vi "FRCts20_Backend_Division_POST.vi"(6 "Message Attributes":T4, 8 "error in (no error)":errorcluster, 10 "Data":string, 11 "Engine_Refnums":T1) -> (0 "error out":errorcluster)   [LabVIEW 2014]
doc: "Creates a new division under a competition. Called by the division/team api, and expects a division location and competition name."
uses:
  Dependencies/Keyed Array/KeyedArray.ctl
  FRCts20_Backend_EngineRefnums.ctl
  INI_Accessor/FRCts20_Backend_INI Controller.lvclass
  Dependencies/AMC/_SubVIs/TypeDefs/Message Queue.ctl
  Dependencies/AMC/_SubVIs/TypeDefs/Message.ctl
  <vilib>/addons/database/Connection.llb/Conn ObjectReference.ctl
  FRCts20_Backend_FGVOperation.ctl
  FRCts20_Backend_API/FRCts20_Backend_API_Division.ctl
  FRCts20_Backend_API/FRCts20_Backend_API_SW.ctl
  FRCts20_Backend_API/FRCts20_Backend_API_Status.ctl
  FRCts20_Backend_Engine.lvlib
  FRCts20_Backend_API/FRCts20_Backend_API.lvlib
  Dependencies/Keyed Array/Tools_KeyedArray.lvlib
  Dependencies/AMC/AMC.lvlib
  <vilib>/addons/database/NI_Database_API.lvlib
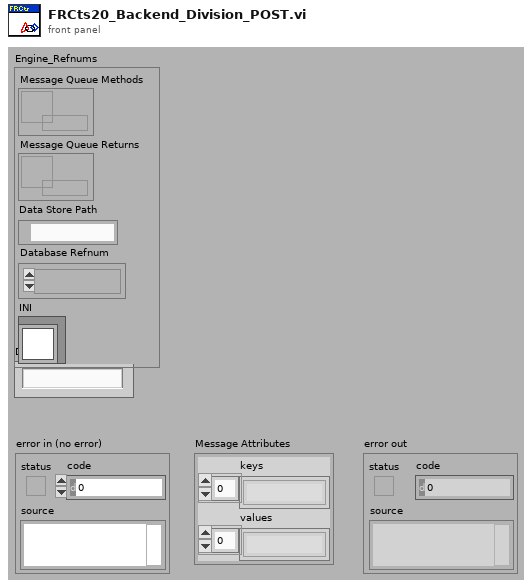
[diagram p1: front panel]
types:
  T1 = typedef "FRCts20_Backend_Engine.lvlib/FRCts20_Backend_EngineRefnums.ctl" = cluster{"Message Queue Methods":T2, "Message Queue Returns":T2, "Data Store Path":path, "Database Refnum":T3, "INI":refnum<class "FRCts20_Backend_INI Controller.lvclass">}
  T2 = typedef "AMC.lvlib/Message Queue.ctl" = refnum<queue>
  T3 = typedef "NI_Database_API.lvlib/Conn ObjectReference.ctl" = refnum<k1>
  T4 = typedef "Tools_KeyedArray.lvlib/KeyedArray.ctl" = cluster{"keys":string[], "values":string[]}
  T5 = typedef "FRCts20_Backend_API.lvlib/FRCts20_Backend_API_Division.ctl" = cluster{"Location":string, "Team":u32[], "APIReturn":string, "RootCmd":enum16{"Issues", "Software", "All"}, "SWType":T6, "Status":T7, "Competition":string}
  T6 = typedef "FRCts20_Backend_API.lvlib/FRCts20_Backend_API_SW.ctl" = string
  T7 = typedef "FRCts20_Backend_API.lvlib/FRCts20_Backend_API_Status.ctl" = enum16{"Open", "In Work", "Closed"}
  T8 = typedef "FRCts20_Backend_Engine.lvlib/FRCts20_Backend_FGVOperation.ctl" = enum16{"Initialize", "EnqueueMessage", "EnqueueDataReturn", "FlushMessage", "FlushDataReturn"}
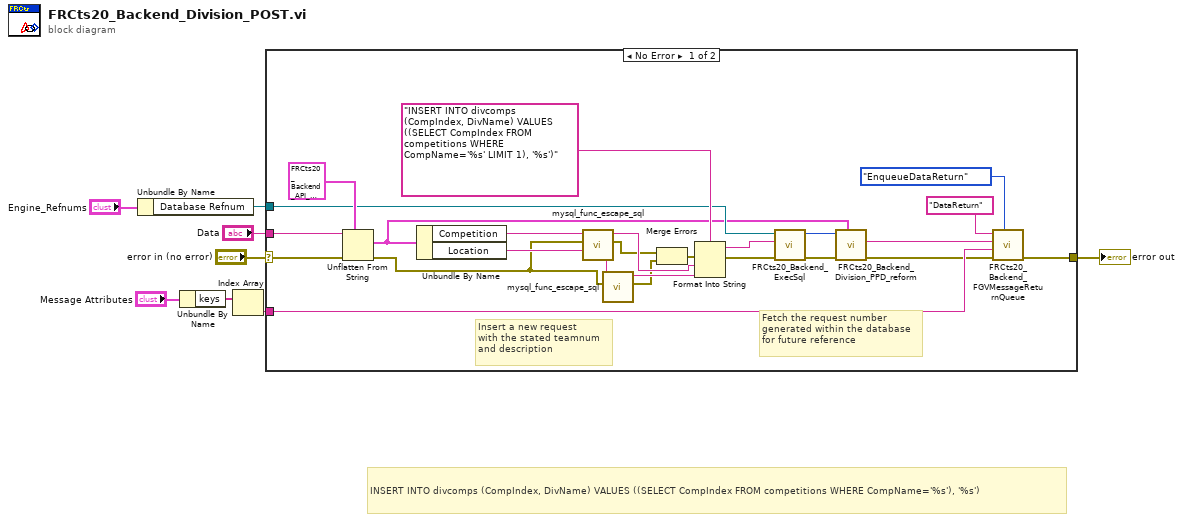
[diagram p0: block diagram]
diagram:
  # "INSERT INTO divcomps (CompIndex, DivName) VALUES ((SELECT CompIndex FROM competitions WHERE CompName='%s'), '%s')"
  n1 = Unbundle By Name("Engine_Refnums") -> ("Database Refnum"=w5:T3)
  n2 = Unbundle By Name("Message Attributes") -> ("keys"=w2:string[])
  n3 = Index Array(array=w2) -> (element=w1:string)  [unwired: 1 in]
  n4 = case shown="No Error" "error in (no error)" {
    selector: "error in (no error)" -> [w29 w33]
    tunnel: [w32 w33] -> w7
    tunnel: w5 -> [w16 _]
    tunnel: "Data" -> [w30 _]
    tunnel: w1 -> [w31 _]
    frame No Error {
      # "Fetch the request number\ngenerated within the database\nfor future reference"
      # "Insert a new request\nwith the stated teamnum\nand description"
      n5 = Unflatten From String(type=T5 {"Location"="", "Team"=[], "APIReturn"="", "RootCmd"=enum."Issues", "SWType"="", "Status"=enum."Open", "Competition"=""} ("Division"), binary string=w30, error in (no error)=w29) -> (value=w9:T5, error out=w10:errorcluster)  [unwired: 2 in, 1 out]
      n6 = Unbundle By Name(w9) -> ("Competition"=w22:string, "Location"=w21:string)
      n7 = call "mysql_func_escape_sql.vi"("error in (no error)"=w10, "sqlin"=w22) -> ("error out"=w12:errorcluster, "escaped"=w19:string)  [unwired: 8 in]
      n8 = call "mysql_func_escape_sql.vi"("error in (no error)"=w10, "sqlin"=w21) -> ("error out"=w11:errorcluster, "escaped"=w20:string)  [unwired: 8 in]
      n9 = Merge Errors(w12, w11) -> (w13:errorcluster)
      n10 = Format Into String(format string="INSERT INTO divcomps (CompIndex, DivName) VALUES ((SELECT CompIndex FROM competitions WHERE CompName='%s' LIMIT 1), '%s')", error in=w13, w19, w20) -> (resulting string=w15:string, error out=w14:errorcluster)  [unwired: 1 in]
      n11 = call "FRCts20_Backend_ExecSql.vi"("error in (no error)"=w14, "format string"=w15, "Refnum in"=w16) -> ("error out"=w17:errorcluster, "rows affected"=w18:i32)  [unwired: 6 in, 1 out]
      n12 = call "FRCts20_Backend_Division_PPD_reform.vi"("Division"=w9, "error in (no error)"=w17, "rows affected"=w18) -> ("error out"=w24:errorcluster, "data string"=w25:string)  [unwired: 7 in]
      n13 = call "FRCts20_Backend_FGVMessageReturnQueue.vi"("Operation"=FRCts20_Backend_FGVOperation."EnqueueDataReturn", "error in (no error)"=w24, "Key"=w31, "Message Value"=w25, "Message Name"="DataReturn") -> ("error out"=w32:errorcluster)  [unwired: 5 in, 1 out]
    }
    frame Error {
    }
  }
  "error out" <- w7
